vi "CameraSerialController_v06.vi"() -> (4 "图像时间戳":u32=16532020 format="%_32g")   [LabVIEW 2015]
uses:
  <vilib>/Instr/_visa.llb/VISA Configure Serial Port (Instr).vi
  MVCAMSDK.dll
  <vilib>/Analysis/NI_AALBase.lvlib
panel:
  in  "转动前进":T1=TRUE
  out "光强图 4":dbl[](graph)
  out "variance 4":dbl caption="方差" format="%0.2f"
  out "光强图 3":dbl[](graph)
  out "variance 3":dbl caption="方差" format="%0.2f"
  out "转动信号曲线":cluster{"Locations":dbl[], "Amplitudes":dbl[]}[](graph)=[{"Locations"=array[750 elements], "Amplitudes"=array[749 elements]}, {"Locations"=[104.38621227921368, 258.3247060234782, 410.71523318402836, 562.6858730022967, 712.7065754646931], "Amplitudes"=[11153.698204083417, 10559.387052180104, 10974.865031894917, 10500.852817232146, 11059.763900010517]}, {"Locations"=[26.787398227992274, 182.39455189327623, 333.5517219531509, 488.1851999460032, 636.5270621135614], "Amplitudes"=[3284.809720018355, 2039.4564261182056, 3638.2587716464914, 3082.2730888167225, 4217.856016996603]}]
  in  "平移回退":T1=TRUE
  in  "转动回退":T1=TRUE
  in  "转动计数":u16
  in  "转动一次脉冲数":u16=20
  in  "平移一次脉冲数":u16=20
  in  "平移计数":u16
  out "variance 2":dbl caption="方差" format="%0.2f"
  in  "flow control (0:none)":u16(ring) caption="流控制（0:无）" items=["无", "XON/XOFF", "RTS/CTS", "XON/XOFF & RTS/CTS", "DTR/DSR", "XON/XOFF & DTR/DSR"]
  in  "stop bits (10: 1 bit)":u16=10 caption="停止位（10: 1位）"
  in  "奇偶 (0:none)":enum16{"None", "Odd", "Even", "Mark", "Space"}(ring) caption="奇偶（0:无）"
  in  "数据比特(默认8)":u16(ring)=8 items=["5"=5, "6"=6, "7"=7, "8"=8]
  in  "波特率(默认9600)":u32=9600
  in  "端口":refnum<visa-resource-name>="COM1"
  in  "开始":T1=TRUE
  out "泰伯距离数值":dbl[](array[numeric])=[15.393849374426454, 15.239052716055017, 15.197063981826837, 15.002070246239633]
  out "Locations":dbl[](array[numeric])=[10.438621227921368, 25.832470602347822, 41.07152331840284, 56.268587300229676, 71.27065754646931] caption="上面图像曲线波峰位置"
  out "平移信号曲线":cluster{"Locations":dbl[], "Amplitudes":dbl[]}[](graph)=[{"Locations"=array[750 elements], "Amplitudes"=array[749 elements]}, {"Locations"=[104.38621227921368, 258.3247060234782, 410.71523318402836, 562.6858730022967, 712.7065754646931], "Amplitudes"=[11153.698204083417, 10559.387052180104, 10974.865031894917, 10500.852817232146, 11059.763900010517]}, {"Locations"=[26.787398227992274, 182.39455189327623, 333.5517219531509, 488.1851999460032, 636.5270621135614], "Amplitudes"=[3284.809720018355, 2039.4564261182056, 3638.2587716464914, 3082.2730888167225, 4217.856016996603]}]
  out "光强图 2":dbl[](graph)
  out "variance":dbl caption="方差" format="%0.2f"
  out "相机图像":T2(plugin-control)
  out "光强图":dbl[](graph)
  in  "自定义分辨率设置":bool
  in  "ROI分辨率":T3
  in  "预设分辨率设置":bool
  in  "预设分辨率":T4(radio)
  out "帧速":u32
  out "帧间耗时\n单位：（0.1ms）":u32
  in  "相机枚举":T5(ring)
  in  "自动曝光模式":bool=TRUE caption="软触发"
  in  "手动曝光模式":bool caption="软触发"
  in  "曝光时间，单位微秒":dbl=11000.0 format="%#_6f"
  in  "硬触发模式":bool caption="软触发"
  in  "软触发模式":bool caption="软触发"
  in  "连续模式":bool caption="软触发"
  in  "软触发一帧":bool caption="软触发"
  in  "读取自定义数据":bool
  out "从相机中读出的字符串(32字节)":string
  in  "写入自定义数据":bool
  in  "要写入相机的字符串(32字节)":string
  in  "拍照":bool
  in  "相机参数":bool=TRUE
  in  "Stop":bool
  in  "激活预览":bool=TRUE
  out "Image":T2(plugin-control)
  # "相机原生分辨率设置"
  # "写入自定义数据"
  # "触发设置"
  # "曝光设置"
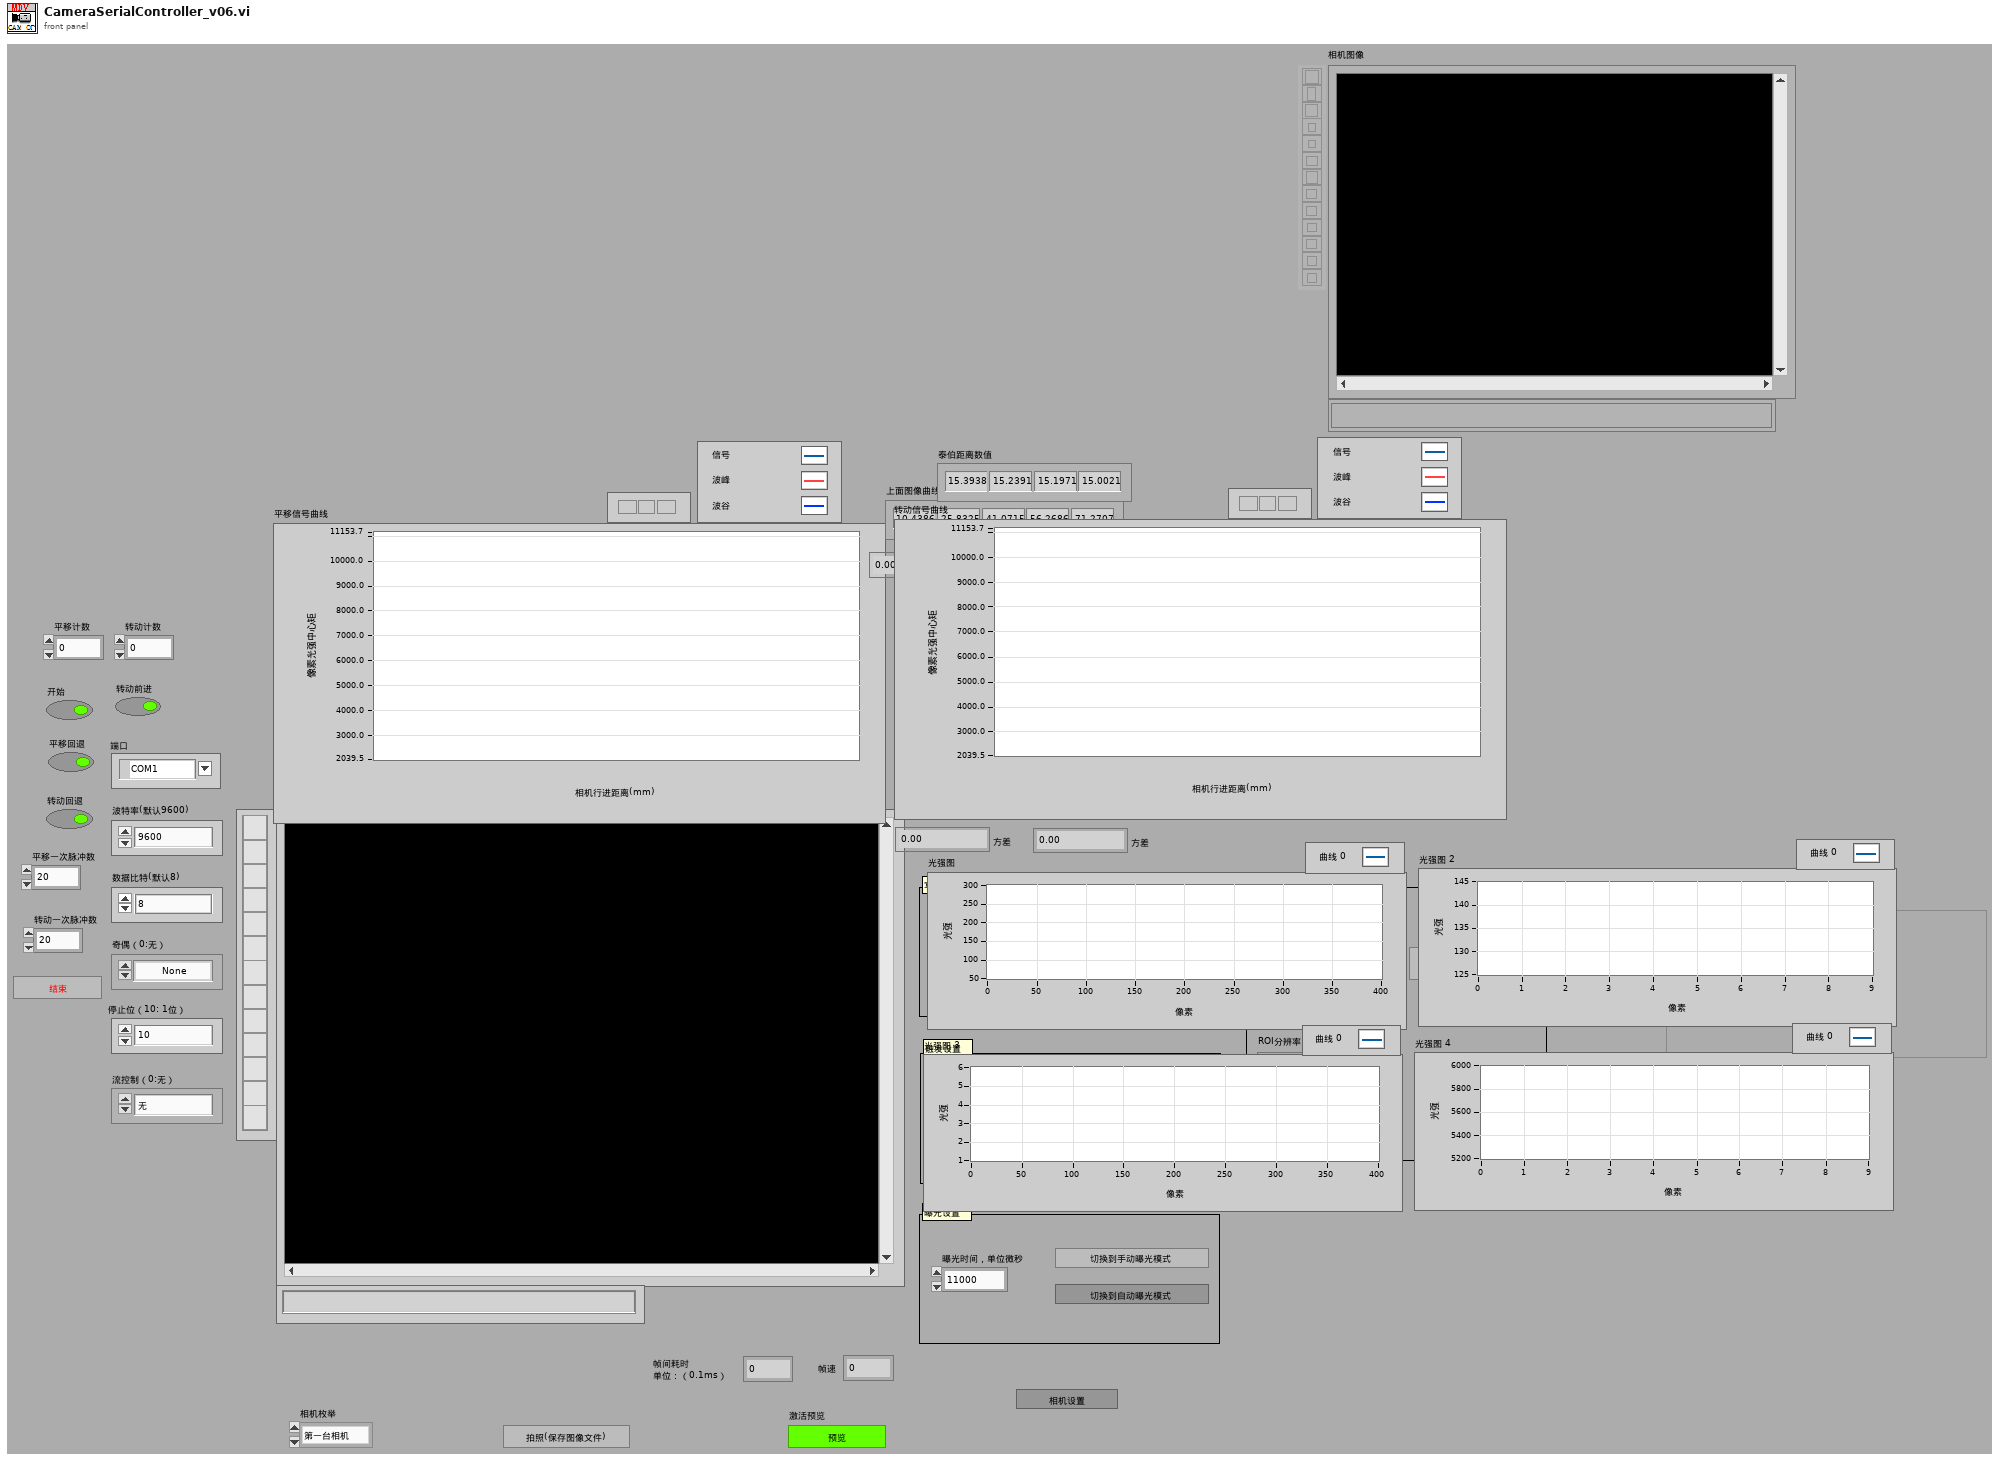
[diagram p1: front panel]
types:
  T1 = typedef "控件 1.ctl" = bool
  T2 = typedef "IMAQ Image.ctl" = refnum<image>
  T3 = cluster{"水平偏移":dbl, "垂直偏移":dbl, "宽度":dbl, "高度":dbl}
  T4 = enum32{"分辨率1", "分辨率2", "分辨率3", "分辨率4", "分辨率5", "分辨率6"}
  T5 = enum16{"第一台相机", "第二台相机", "第三台相机", "第四台相机", "第五台相机"}
  T6 = typedef "Image Type" = u32
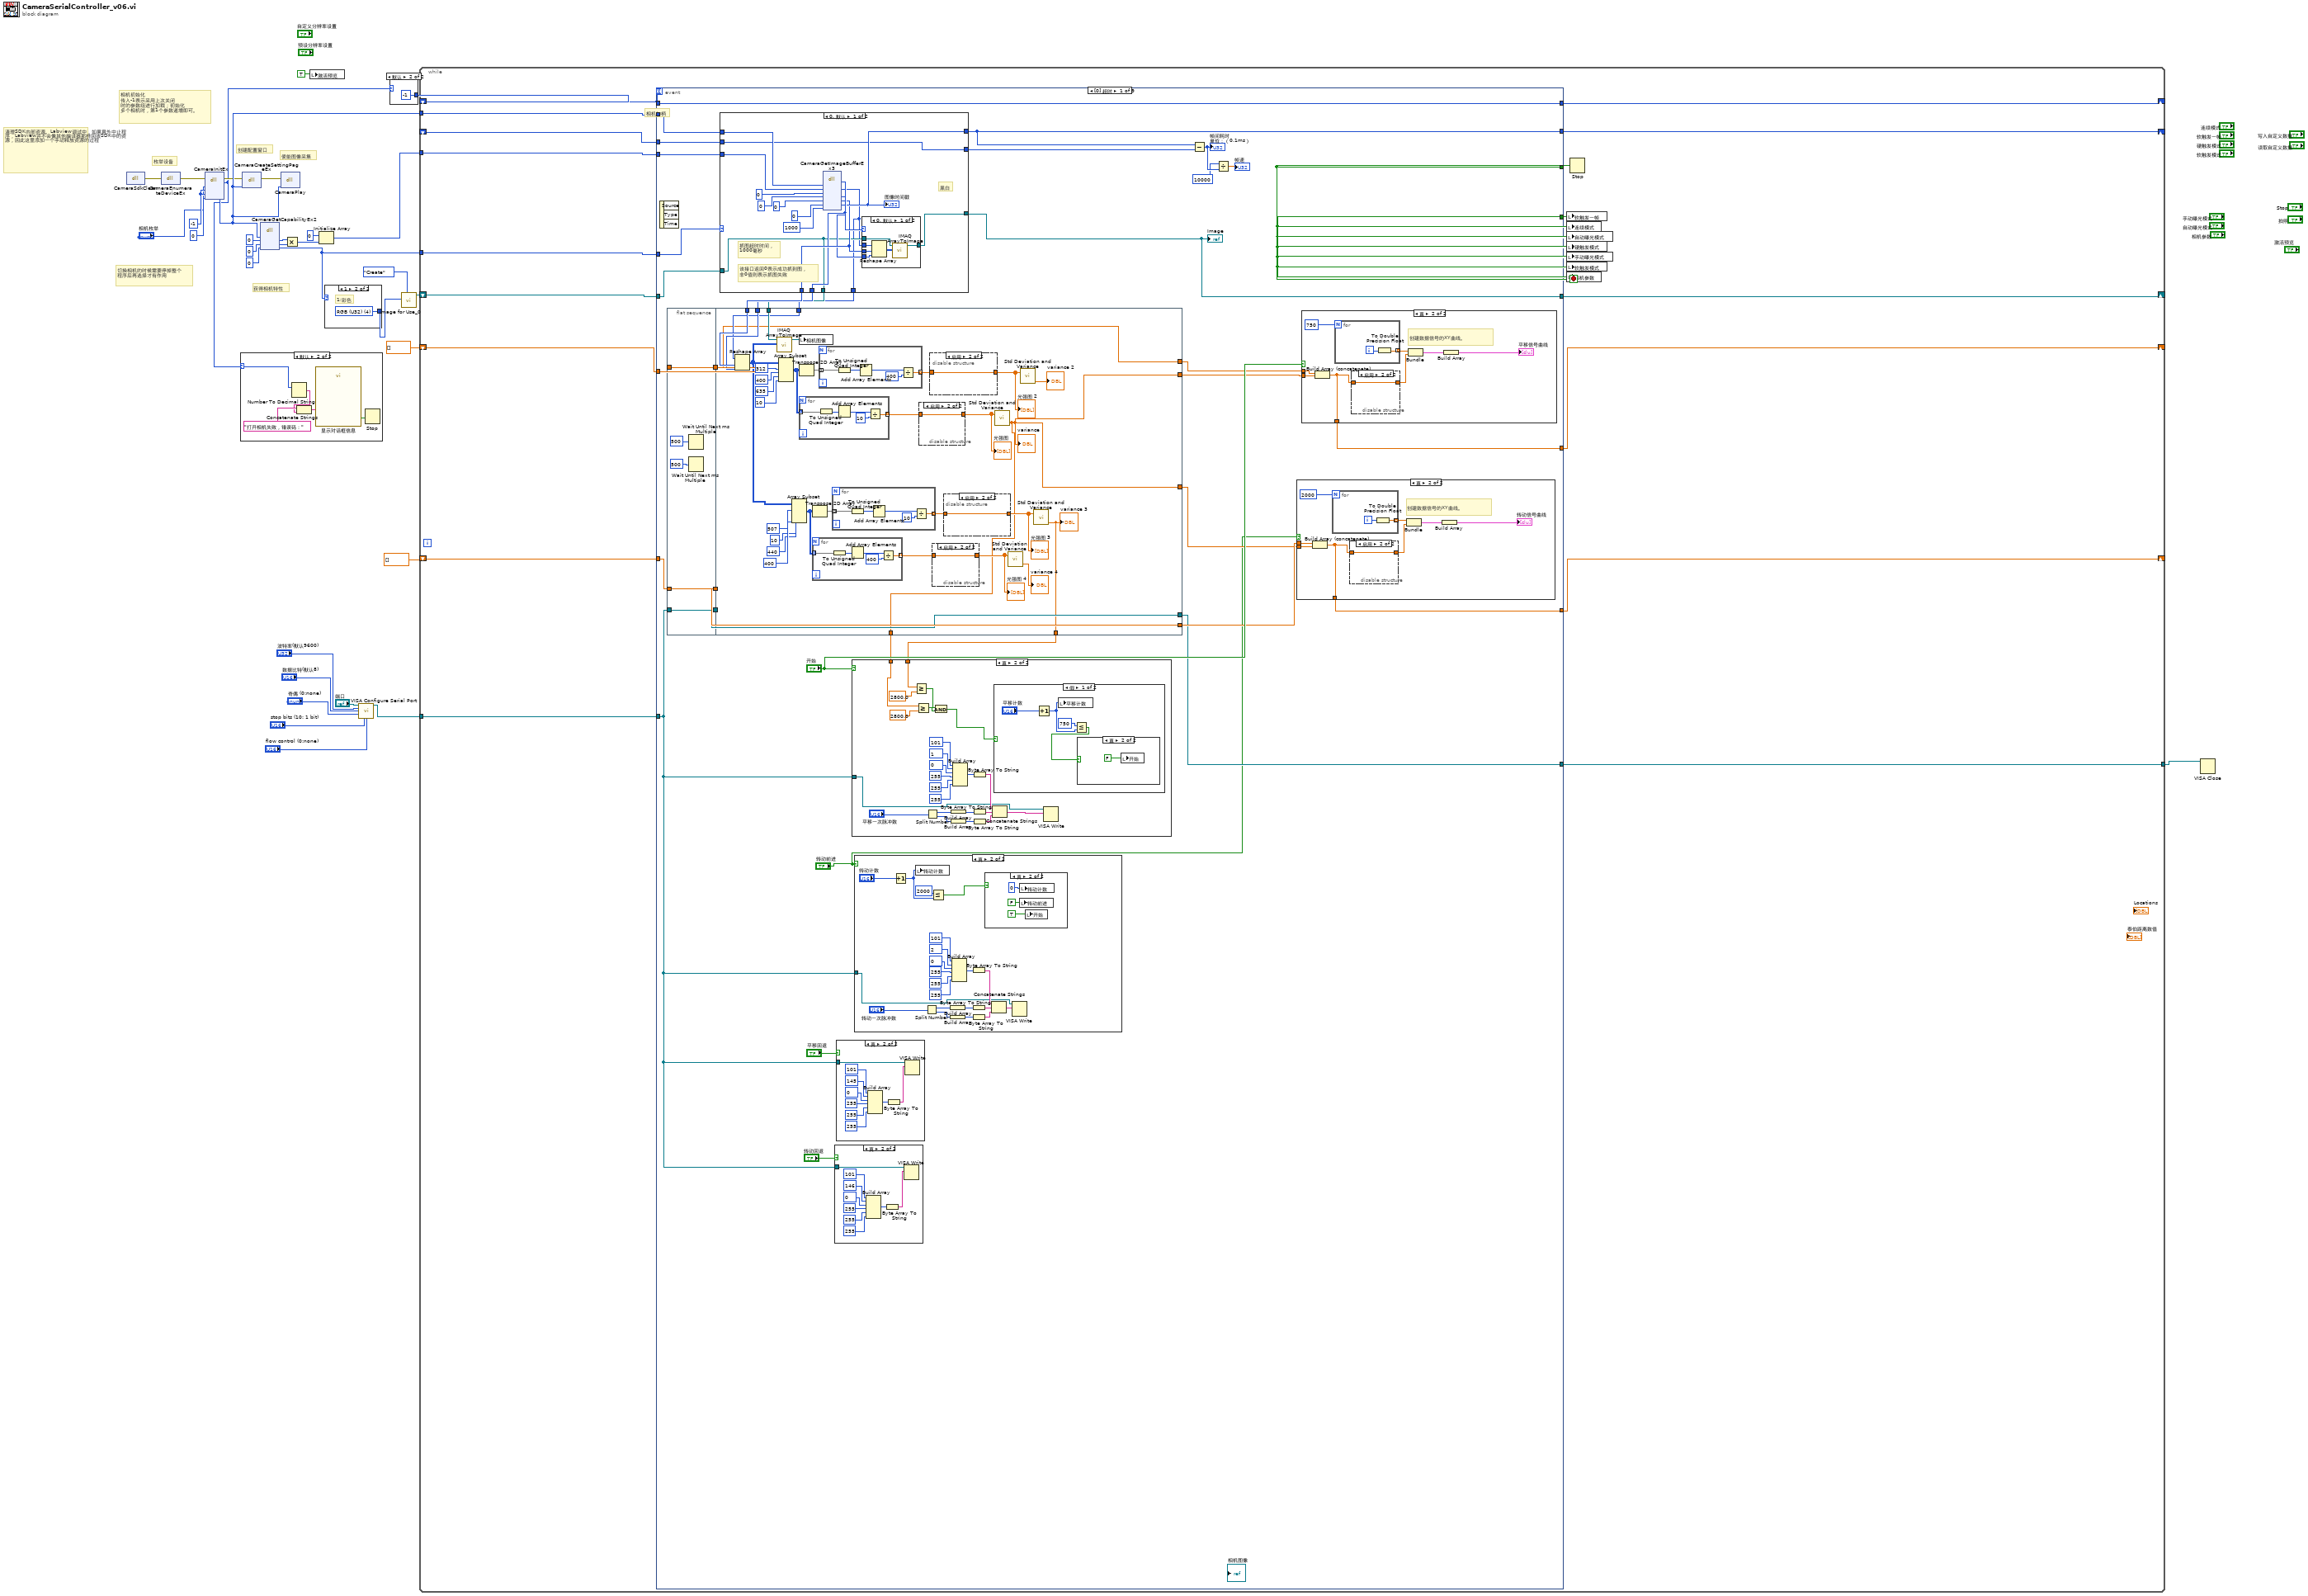
[diagram p0: block diagram]
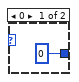
[diagram p2: hidden frame]
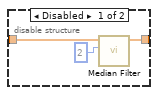
[diagram p4: hidden frame]
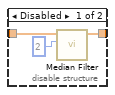
[diagram p5: hidden frame]
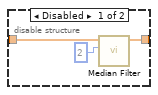
[diagram p6: hidden frame]
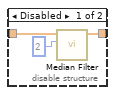
[diagram p7: hidden frame]
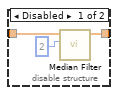
[diagram p9: hidden frame]
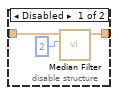
[diagram p11: hidden frame]
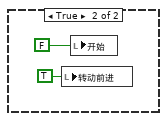
[diagram p18: hidden frame]
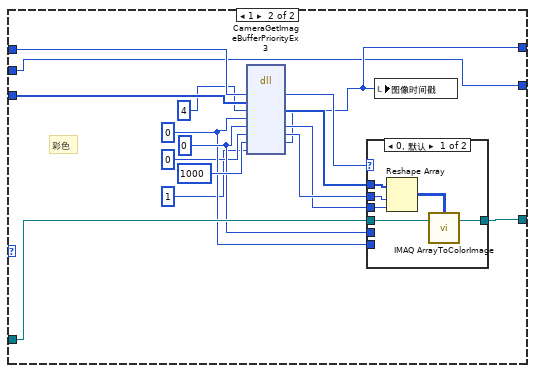
[diagram p20: hidden frame]
diagram:
  w30 = -1
  # "切换相机的时候需要停掉整个\n程序后再选择才有作用"
  # "清理SDK内部资源。Labview调试中，如果意外中止程序，Labview并不会像其他编译器那样回收SDK中的资源，因此这里添加一个手动释放资源的过程"
  # "使能图像采集"
  # "获得相机特性"
  # "创建配置窗口"
  # "相机初始化\n传入-1表示采用上次关闭\n时的参数组进行加载；初始化\n多个相机时，第1个参数递增即可。"
  # "枚举设备"
  n1 = dll-call lib="MVCAMSDK.dll" fn="CameraSdkClean"() -> (error out=w31:errorcluster)  [unwired: 4 in, 1 out]
  n2 = dll-call lib="MVCAMSDK.dll" fn="CameraEnumerateDeviceEx"(error in=w31) -> (error out=w28:errorcluster)  [unwired: 3 in, 1 out]
  n3 = dll-call lib="MVCAMSDK.dll" fn="CameraInitEx"(error in=w28, "相机索引值"="相机枚举", "参数加载方式"=w30, "要加载的参数组索引"=w30, "相机句柄"=0) -> (error out=w17:errorcluster, "返回类型"=w12:i32, "相机句柄"=w19:i32)  [unwired: 5 in, 1 out]
  n4 = case shown="默认" w12 {
    selector: w12 -> [_ w37]
    frame 0 {
    }
    frame Default {
      n5 = Number To Decimal String(number=w37) -> (decimal integer string=w34:string)  [unwired: 1 in]
      n6 = Concatenate Strings("打开相机失败，错误码：" ("字符串"), w34) -> (w36:string)
      n7 = call "显示对话框信息"("Message"=w36) -> ("结束"=w38:bool)  [unwired: 9 in, 1 out]
      n8 = Stop(stop? (T)=w38) -> ()
    }
  }
  n9 = dll-call lib="MVCAMSDK.dll" fn="CameraCreateSettingPageEx"(error in=w17, "相机句柄"=w19) -> (error out=w20:errorcluster)  [unwired: 4 in, 1 out]
  n10 = dll-call lib="MVCAMSDK.dll" fn="CameraGetCapabilityEx2"("相机句柄"=w19, "图像最大宽度"=0, "图像最大高度"=0, "是否是彩色相机(返回0:黑白;1:彩色)"=0) -> ("图像最大宽度"=w22:i32, "图像最大高度"=w21:i32, "是否是彩色相机(返回0:黑白;1:彩色)"=w16:i32)  [unwired: 5 in, 2 out]
  n11 = dll-call lib="MVCAMSDK.dll" fn="CameraPlay"(error in=w20, "相机句柄"=w19) -> ()  [unwired: 4 in, 2 out]
  n12 = Multiply(x=w22, y=w21) -> (x*y=w26:i32)
  n13 = local write "激活预览"(TRUE ("激活预览")) -> ()
  n14 = Initialize Array(0, w26) -> (w18:i32[])
  n15 = case shown="1" w16 {
    tunnel: [_ w39] -> w32
    frame 0, Default {
      # "0:黑白;"
    }
    frame 1 {
      w39 = T6 4 items=["Grayscale (U8)", "Grayscale (I16)", "Grayscale (SGL)", "Complex (CSG)", "RGB (U32)", "HSL (U32)", "RGB (U64)", "Grayscale (U16)"] ("Image Type")
      # "1:彩色"
    }
  }
  n16 = call-poly "VISA Configure Serial Port"("VISA resource name"="端口", "baud rate (9600)"="波特率(默认9600)", "data bits (8)"="数据比特(默认8)", "parity (0:none)"="奇偶 (0:none)", "stop bits (10: 1 bit)"="stop bits (10: 1 bit)", "flow control (0:none)"="flow control (0:none)") -> ("VISA resource name out"=w4:refnum<visa-resource-name>)  [unwired: 8 in, 1 out]
  n17 = case shown="默认" w12 {
    tunnel: [0 -1] -> w11
    frame 0 {
    }
    frame Default {
    }
  }
  n18 = call "Image for Use_0.vi"("Command"=enum16{"Create", "Use", "Copy in", "Dispose"}."Create", "Image Type"=w32) -> ("Image out"=w15:T2)  [unwired: 8 in, 1 out]
  n19 = while {
    tunnel: w19 -> [w55]
    tunnel: w18 -> [w57]
    tunnel: w16 -> [w58]
    shift-right: [w54] -> _
    shift-left: w11 -> [w53]
    shift-right: [w51] -> _
    shift-left: w15 -> [w56]
    shift-right: [w50] -> _
    shift-left: _ -> [w49]
    tunnel: w4 -> [w47]
    tunnel: [w46] -> w3
    shift-right: [w44] -> _
    shift-left: dbl[] [] -> [w45]
    shift-right: [w43] -> _
    shift-left: dbl[] [] -> [w42]
    stop <- w48 stop-if-true
    # "相机句柄"
    n20 = event shown="[0] 超时" {
      selector: _ -> [_ _ _ _ _ _ _ _ _]
      dyn-events: _ -> [_ _ _ _ _ _ _ _ _]
      timeout: w53 -> [_ _ _ _ _ _ _ _ _]
      tunnel: [_ _ _ _ _ _ _ _ TRUE] -> w48
      tunnel: w57 -> [w92 _ _ _ _ _ _ _ _]
      tunnel: w58 -> [w91 _ _ _ _ _ _ _ _]
      tunnel: w55 -> [w93 _ w324 w342 w357 _ w371 w394 w474]
      tunnel: w56 -> [w90 w317 w323 w341 w356 w361 w370 w396 w472]
      tunnel: [w89 w318 w325 w343 w358 w362 w372 w397 w475] -> w54
      tunnel: w53 -> [w89 _ w325 w343 w358 w362 w372 w397 w475]
      tunnel: [_ _ _ _ _ _ _ _ FALSE] -> w52
      tunnel: [w88 w317 w323 w341 w356 w361 w370 w396 w472] -> w51
      tunnel: [w85 w316 w322 w340 w355 w360 w369 w388 w471] -> w50
      tunnel: w49 -> [w87 w316 w322 w340 w355 w360 w369 w388 w471]
      tunnel: w47 -> [w66 _ _ _ _ _ _ _ _]
      tunnel: [w65 _ _ _ _ _ _ _ _] -> w46
      tunnel: w45 -> [w72 _ _ _ _ _ _ _ _]
      tunnel: [w74 _ _ _ _ _ _ _ _] -> w44
      tunnel: [w73 _ _ _ _ _ _ _ _] -> w43
      tunnel: w42 -> [w68 _ _ _ _ _ _ _ _]
      event Timeout {
        n21 = event-data() -> ()  [unwired: 1 in, 3 out]
        n22 = flat-sequence {
          tunnel: w72 -> [w98]
          tunnel: [w98] -> w71
          tunnel: [w95] -> w69
          tunnel: w68 -> [w95]
          tunnel: [w94] -> w67
          tunnel: w66 -> [w94]
          tunnel: w81 -> [w130]
          tunnel: w80 -> [w129]
          tunnel: w79 -> [w128]
          tunnel: w78 -> [w127]
          tunnel: [w99] -> w63
          tunnel: [w116] -> w62
          tunnel: w71 -> [w116]
          tunnel: [w115] -> w70
          tunnel: w69 -> [w115]
          tunnel: [w114] -> w65
          tunnel: w67 -> [w114]
          tunnel: [w99] -> w64
          tunnel: [w100] -> w61
          tunnel: [w99] -> w60
          frame #0 {
            n23 = Wait Until Next ms Multiple(millisecond multiple=u32 500 ("毫秒倍数")) -> ()  [unwired: 1 out]
            n24 = Wait Until Next ms Multiple(millisecond multiple=u32 500 ("毫秒倍数")) -> ()  [unwired: 1 out]
          }
          frame #1 {
            n25 = Reshape Array(w127, w130, w129) -> (w101:u8[][])
            n26 = call "IMAQ ArrayToImage"("Image Pixels (U8)"=w101, "Image"=w128) -> ("Image Out"=w131:T2)  [unwired: 8 in, 1 out]
            n27 = Array Subset(array=w101, index (row)=312 ("索引"), length (row)=400 ("长度"), index (col)=635 ("长度"), length (col)=10 ("索引")) -> (w117:u8[][])
            n28 = Array Subset(array=w101, index (row)=507 ("索引"), length (row)=10 ("长度"), index (col)=440 ("长度"), length (col)=400 ("索引")) -> (w112:u8[][])
            n29 = local write "相机图像"(w131) -> ()
            n30 = Transpose 2D Array(2D array=w117) -> (transposed array=w124:u8[][])
            n31 = for {
              tunnel: w117 -> [w162] mode=indexing
              tunnel: [w160] -> w126 mode=indexing
              n32 = To Unsigned Quad Integer(1:w162) -> (0:w161:u64[])
              n33 = Add Array Elements(numeric array=w161) -> (sum=w163:u64)
              n34 = Divide(x=w163, y=u64 10) -> (x/y=w160:dbl)
            }
            n35 = Transpose 2D Array(2D array=w112) -> (transposed array=w105:u8[][])
            n36 = for {
              tunnel: w112 -> [w144] mode=indexing
              tunnel: [w142] -> w103 mode=indexing
              n37 = To Unsigned Quad Integer(1:w144) -> (0:w143:u64[])
              n38 = Add Array Elements(numeric array=w143) -> (sum=w145:u64)
              n39 = Divide(x=w145, y=u64 400) -> (x/y=w142:dbl)
            }
            n40 = for {
              tunnel: w124 -> [w153] mode=indexing
              tunnel: [w151] -> w125 mode=indexing
              n41 = To Unsigned Quad Integer(1:w153) -> (0:w152:u64[])
              n42 = Add Array Elements(numeric array=w152) -> (sum=w154:u64)
              n43 = Divide(x=w154, y=u64 400) -> (x/y=w151:dbl)
            }
            n44 = for {
              tunnel: w105 -> [w135] mode=indexing
              tunnel: [w133] -> w104 mode=indexing
              n45 = To Unsigned Quad Integer(1:w135) -> (0:w134:u64[])
              n46 = Add Array Elements(numeric array=w134) -> (sum=w136:u64)
              n47 = Divide(x=w136, y=u64 10) -> (x/y=w133:dbl)
            }
            n48 = disable-structure shown="启用" {
              disable-tunnel: w126 -> [w166 w167]
              disable-tunnel: [w164 w167] -> w123
              frame Disabled {
                n49 = call <vilib>:"Median Filter.vi"("left rank"=2, "X"=w166) -> ("Filtered X"=w164:dbl[])  [unwired: 8 in, 1 out]
              }
              frame Enabled {
              }
            }
            "光强图" <- w123
            n50 = disable-structure shown="启用" {
              disable-tunnel: w125 -> [w157 w158]
              disable-tunnel: [w155 w158] -> w122
              frame Disabled {
                n51 = call <vilib>:"Median Filter.vi"("left rank"=2, "X"=w157) -> ("Filtered X"=w155:dbl[])  [unwired: 8 in, 1 out]
              }
              frame Enabled {
              }
            }
            "光强图 2" <- w122
            n52 = disable-structure shown="启用" {
              disable-tunnel: w103 -> [w148 w149]
              disable-tunnel: [w146 w149] -> w106
              frame Disabled {
                n53 = call <vilib>:"Median Filter.vi"("left rank"=2, "X"=w148) -> ("Filtered X"=w146:dbl[])  [unwired: 8 in, 1 out]
              }
              frame Enabled {
              }
            }
            "光强图 4" <- w106
            n54 = disable-structure shown="启用" {
              disable-tunnel: w104 -> [w139 w140]
              disable-tunnel: [w137 w140] -> w107
              frame Disabled {
                n55 = call <vilib>:"Median Filter.vi"("left rank"=2, "X"=w139) -> ("Filtered X"=w137:dbl[])  [unwired: 8 in, 1 out]
              }
              frame Enabled {
              }
            }
            "光强图 3" <- w107
            n56 = call <vilib>:"Std Deviation and Variance.vi"("X"=w123) -> ("variance"=w99:dbl)  [unwired: 1 in, 2 out]
            "variance" <- w99
            n57 = call <vilib>:"Std Deviation and Variance.vi"("X"=w106) -> ("variance"=→"variance 4":dbl)  [unwired: 1 in, 2 out]
            n58 = call <vilib>:"Std Deviation and Variance.vi"("X"=w122) -> ("variance"=→"variance 2":dbl)  [unwired: 1 in, 2 out]
            n59 = call <vilib>:"Std Deviation and Variance.vi"("X"=w107) -> ("variance"=w100:dbl)  [unwired: 1 in, 2 out]
            "variance 3" <- w100
          }
        }
        n60 = case shown="0, 默认" w91 {
          tunnel: w92 -> [w285 w308]
          tunnel: w90 -> [w272 w307]
          tunnel: w93 -> [w277 w306]
          tunnel: [w278 w296] -> w88
          tunnel: [w276 w295] -> w85
          tunnel: w87 -> [w275 w294]
          tunnel: [w275 w294] -> w86
          tunnel: [w274 _] -> w81
          tunnel: [w273 _] -> w80
          tunnel: [w272 _] -> w79
          tunnel: [w271 _] -> w78
          frame 0, Default {
            # "黑白"
            # "该接口返回0表示成功抓到图，\n非0值则表示抓图失败"
            # "抓图超时时间，\n1000毫秒"
            n61 = dll-call lib="MVCAMSDK.dll" fn="CameraGetImageBufferEx3"("相机句柄"=w277, "图像数据缓冲区"=w285, "图像输出格式(0:8位灰度;1:24位彩色;2:32位彩色，3：BGR24彩色 4：BGRA32位彩色)"=0, "图像宽度"=0, "图像高度"=0, "时间戳(单位为100微秒)"=0, "抓图超时时间(毫秒)"=1000) -> ("返回类型"=w280:i32, "图像数据缓冲区"=w271:u8[], "图像宽度"=w273:i32, "图像高度"=w274:i32, "时间戳(单位为100微秒)"=w276:u32)  [unwired: 6 in, 2 out]
            "图像时间戳" <- w276
            n62 = case shown="0, 默认" w280 {
              tunnel: w271 -> [w291 _]
              tunnel: w272 -> [w288 w292]
              tunnel: w274 -> [w290 _]
              tunnel: w273 -> [w289 _]
              tunnel: [w286 w292] -> w278
              frame 0, Default {
                n63 = Reshape Array(w291, w290, w289) -> (w287:u8[][])
                n64 = call "IMAQ ArrayToImage"("Image Pixels (U8)"=w287, "Image"=w288) -> ("Image Out"=w286:T2)  [unwired: 8 in, 1 out]
              }
              frame -12 {
              }
            }
          }
          frame 1 {
            w298 = 0
            w299 = 0
            # "彩色"
            n65 = dll-call lib="MVCAMSDK.dll" fn="CameraGetImageBufferPriorityEx3"("相机句柄"=w306, "图像数据缓冲区"=w308, "图像输出格式(0:8位灰度;1:24位彩色;2:32位彩色)"=4, "图像宽度"=w298, "图像高度"=w299, "时间戳（单位为100微秒）"=0, "抓图超时时间(毫秒)"=1000, "取图优先级(0: 取最旧   1:取最新)"=1) -> ("返回类型"=w300:i32, "图像数据缓冲区"=w303:u32[], "图像宽度"=w301:i32, "图像高度"=w302:i32, "时间戳（单位为100微秒）"=w295:u32)  [unwired: 7 in, 2 out]
            n66 = case shown="0, 默认" w300 {
              tunnel: w303 -> [w313 _]
              tunnel: w307 -> [w312 w315]
              tunnel: w302 -> [w311 _]
              tunnel: w301 -> [w310 _]
              tunnel: w299 -> [_ _]
              tunnel: w298 -> [_ _]
              tunnel: [w309 w315] -> w296
              frame 0, Default {
                n67 = Reshape Array(w313, w311, w310) -> (w314:u32[][])
                n68 = call "IMAQ ArrayToColorImage"("Image Pixels (U32)"=w314, "Image"=w312) -> ("Image Out"=w309:T2)  [unwired: 3 in, 1 out]
              }
              frame -12 {
              }
            }
            n69 = local write "图像时间戳"(w295) -> ()
          }
        }
        "Image" <- w88
        n70 = case shown="真" "转动回退" {
          tunnel: w66 -> [_ w199]
          frame False {
          }
          frame True {
            n71 = Build Array(101, 146, 0, 255, 255, 255) -> (w200:i32[])
            n72 = Byte Array To String(unsigned byte array=w200) -> (string=w198:string)
            n73 = VISA Write(VISA resource name=w199, write buffer=w198) -> ()  [unwired: 1 in, 3 out]
          }
        }
        n74 = case shown="真" "平移回退" {
          tunnel: w66 -> [_ w208]
          frame False {
          }
          frame True {
            n75 = Build Array(101, 145, 0, 255, 255, 255) -> (w209:i32[])
            n76 = Byte Array To String(unsigned byte array=w209) -> (string=w207:string)
            n77 = VISA Write(VISA resource name=w208, write buffer=w207) -> ()  [unwired: 1 in, 3 out]
          }
        }
        n78 = case shown="真" "开始" {
          tunnel: w66 -> [_ w248]
          tunnel: w61 -> [_ w246]
          tunnel: w60 -> [_ w245]
          frame False {
          }
          frame True {
            n79 = Greater Or Equal?(x=w246, y=2800.0) -> (x >= y?=w242:bool)
            n80 = Greater Or Equal?(x=w245, y=2800.0) -> (x >= y?=w241:bool)
            n81 = Split Number(x="平移一次脉冲数") -> (hi(x)=w256:u8, lo(x)=w255:u8)
            n82 = And(x=w242, y=w241) -> (x .and. y?=w240:bool)
            n83 = Build Array(w256) -> (w254:u8[])
            n84 = Build Array(w255) -> (w253:u8[])
            n85 = Build Array(101, 1, 0, 255, 255, 255) -> (w252:i32[])
            n86 = Byte Array To String(unsigned byte array=w252) -> (string=w251:string)
            n87 = Byte Array To String(unsigned byte array=w254) -> (string=w250:string)
            n88 = Byte Array To String(unsigned byte array=w253) -> (string=w249:string)
            n89 = Concatenate Strings(w251, w250, w249) -> (w247:string)
            n90 = case shown="假" w240 {
              frame False {
                n91 = Increment(x="平移计数") -> (x+1=w265:u16)
                n92 = local write "平移计数"(w265) -> ()
                n93 = Less Or Equal?(x=750, y=w265) -> (x <= y?=w264:bool)
                n94 = case shown="真" w264 {
                  frame False {
                  }
                  frame True {
                    n95 = local write "开始"(T1 FALSE ("平移前进")) -> ()
                  }
                }
              }
              frame True {
                n96 = local write "转动前进"(T1 TRUE ("平移前进")) -> ()
                n97 = local write "开始"(T1 FALSE ("平移前进")) -> ()
              }
            }
            n98 = VISA Write(VISA resource name=w248, write buffer=w247) -> ()  [unwired: 1 in, 3 out]
          }
        }
        n99 = case shown="真" "转动前进" {
          tunnel: w66 -> [_ w220]
          frame False {
          }
          frame True {
            n100 = Increment(x="转动计数") -> (x+1=w218:u16)
            n101 = local write "转动计数"(w218) -> ()
            n102 = Split Number(x="转动一次脉冲数") -> (hi(x)=w228:u8, lo(x)=w227:u8)
            n103 = Less Or Equal?(x=2000, y=w218) -> (x <= y?=w230:bool)
            n104 = Build Array(w228) -> (w226:u8[])
            n105 = Build Array(w227) -> (w225:u8[])
            n106 = Build Array(101, 2, 0, 255, 255, 255) -> (w224:i32[])
            n107 = Byte Array To String(unsigned byte array=w224) -> (string=w223:string)
            n108 = Byte Array To String(unsigned byte array=w226) -> (string=w222:string)
            n109 = Byte Array To String(unsigned byte array=w225) -> (string=w221:string)
            n110 = case shown="真" w230 {
              frame False {
              }
              frame True {
                n111 = local write "转动前进"(T1 FALSE ("平移前进")) -> ()
                n112 = local write "转动计数"(u16 0 ("平移计数")) -> ()
                n113 = local write "开始"(T1 TRUE ("平移前进")) -> ()
              }
            }
            n114 = Concatenate Strings(w223, w222, w221) -> (w217:string)
            n115 = VISA Write(VISA resource name=w220, write buffer=w217) -> ()  [unwired: 1 in, 3 out]
          }
        }
        n116 = Subtract(x=w85, y=w86) -> (x-y=w84:u32)
        "帧间耗时\n单位：（0.1ms）" <- w84
        n117 = Divide(x=u32 10000 ("帧间耗时"), y=w84) -> (x/y=→"帧速":dbl)
        n118 = case shown="真" "转动前进" {
          tunnel: w64 -> [_ w171]
          tunnel: w70 -> [w168 w170]
          tunnel: [w168 w169] -> w73
          frame False {
          }
          frame True {
            # "创建数据信号的XY曲线。"
            n119 = Build Array (concatenate)(w170, w171) -> (w169:dbl[])
            n120 = for {
              N: i64 2000 ("数值") -> [_]
              tunnel: [w177] -> w173 mode=indexing
              i -> [w178]
              n121 = To Double Precision Float(number=w178) -> (double precision float=w177:dbl)
            }
            n122 = disable-structure shown="启用" {
              disable-tunnel: w169 -> [w180 w182]
              disable-tunnel: [w179 w182] -> w174
              frame Disabled {
                n123 = call <vilib>:"Median Filter.vi"("left rank"=2, "X"=w180) -> ("Filtered X"=w179:dbl[])  [unwired: 8 in, 1 out]
              }
              frame Enabled {
              }
            }
            n124 = Bundle(w173, w174) -> (w176:cluster{dbl[], dbl[]})  [unwired: 1 in]
            n125 = Build Array(w176) -> (→"转动信号曲线":cluster{dbl[], dbl[]}[])
          }
        }
        n126 = case shown="真" "开始" {
          tunnel: w62 -> [w183 w185]
          tunnel: w63 -> [_ w186]
          tunnel: [w183 w184] -> w74
          frame False {
          }
          frame True {
            # "创建数据信号的XY曲线。"
            n127 = Build Array (concatenate)(w185, w186) -> (w184:dbl[])
            n128 = for {
              N: i64 750 ("数值") -> [_]
              tunnel: [w192] -> w190 mode=indexing
              i -> [w193]
              n129 = To Double Precision Float(number=w193) -> (double precision float=w192:dbl)
            }
            n130 = disable-structure shown="启用" {
              disable-tunnel: w184 -> [w195 w197]
              disable-tunnel: [w194 w197] -> w189
              frame Disabled {
                n131 = call <vilib>:"Median Filter.vi"("left rank"=2, "X"=w195) -> ("Filtered X"=w194:dbl[])  [unwired: 8 in, 1 out]
              }
              frame Enabled {
              }
            }
            n132 = Bundle(w190, w189) -> (w187:cluster{dbl[], dbl[]})  [unwired: 1 in]
            n133 = Build Array(w187) -> (→"平移信号曲线":cluster{dbl[], dbl[]}[])
          }
        }
      }
      event "激活预览": Value Change {
        n134 = event-data() -> ("NewVal"=w319:bool)  [unwired: 1 in, 5 out]
        n135 = case shown="真" w319 {
          tunnel: [-1 0] -> w318
          frame False {
          }
          frame True {
          }
        }
      }
      event "连续模式", "软触发一帧", "硬触发模式", "软触发模式": Value Change {
        n136 = event-data() -> ("CtlRef"=w327:refnum<vi>)  [unwired: 1 in, 5 out]
        n137 = control-ref of="连续模式"() -> (w329:refnum<vi>)
        n138 = control-ref of="硬触发模式"() -> (w330:refnum<vi>)
        n139 = control-ref of="软触发模式"() -> (w331:refnum<vi>)
        n140 = control-ref of="软触发一帧"() -> (w332:refnum<vi>)
        n141 = Build Array ("创建数组")(w329, w330, w331, w332) -> (w328:refnum<vi>[])
        n142 = Search 1D Array(1D array=w328, element=w327) -> (index of element=w326:i32)  [unwired: 1 in]
        n143 = case shown="1" w326 {
          tunnel: w324 -> [w333 w335 w337 w339]
          frame 0, Default {
            # "连续模式"
            n144 = dll-call lib="MVCAMSDK.dll" fn="CameraSetTriggerMode"("相机句柄"=w333, "模式"=0) -> ()  [unwired: 6 in, 2 out]
          }
          frame 1 {
            # "硬触发模式"
            n145 = dll-call lib="MVCAMSDK.dll" fn="CameraSetTriggerMode"("相机句柄"=w335, "模式"=2) -> ()  [unwired: 6 in, 2 out]
          }
          frame 2 {
            # "软触发模式"
            n146 = dll-call lib="MVCAMSDK.dll" fn="CameraSetTriggerMode"("相机句柄"=w337, "模式"=1) -> ()  [unwired: 6 in, 2 out]
          }
          frame 3 {
            # "软触发一帧"
            n147 = dll-call lib="MVCAMSDK.dll" fn="CameraSoftTrigger"("相机句柄"=w339) -> ()  [unwired: 5 in, 2 out]
          }
        }
      }
      event "手动曝光模式", "自动曝光模式": Value Change {
        n148 = event-data() -> ("CtlRef"=w346:refnum<vi>)  [unwired: 1 in, 5 out]
        n149 = control-ref of="自动曝光模式"() -> (w344:refnum<vi>)
        n150 = control-ref of="手动曝光模式"() -> (w347:refnum<vi>)
        n151 = Build Array ("创建数组")(w347, w344) -> (w348:refnum<vi>[])
        n152 = Search 1D Array(1D array=w348, element=w346) -> (index of element=w345:i32)  [unwired: 1 in]
        n153 = case shown="0, 默认" w345 {
          tunnel: w342 -> [w349 w353]
          frame 0, Default {
            # "手动曝光模式"
            n154 = dll-call lib="MVCAMSDK.dll" fn="CameraSetAeState"("相机句柄"=w349, "曝光模式(0手动，1自动)"=0) -> (error out=w352:errorcluster)  [unwired: 6 in, 1 out]
            n155 = dll-call lib="MVCAMSDK.dll" fn="CameraSetExposureTime"(error in=w352, "相机句柄"=w349, "曝光时间，单位微秒"="曝光时间，单位微秒") -> ()  [unwired: 5 in, 2 out]
          }
          frame 1 {
            # "自动曝光模式"
            n156 = dll-call lib="MVCAMSDK.dll" fn="CameraSetAeState"("相机句柄"=w353, "曝光模式(0手动，1自动)"=1) -> ()  [unwired: 6 in, 2 out]
          }
        }
      }
      event "相机参数": Value Change {
        n157 = event-data() -> ()  [unwired: 1 in, 6 out]
        n158 = dll-call lib="MVCAMSDK.dll" fn="CameraShowSettingPage"("相机句柄"=w357, "状态"=TRUE) -> ()  [unwired: 6 in, 2 out]
      }
      event "拍照": Value Change {
        n159 = event-data() -> ()  [unwired: 1 in, 6 out]
        n160 = local read "Image"() -> (w363:T2)
        n161 = Format Date/Time String(time format string (%c)="%Y-%m-%d %H：%M：%S.bmp ") -> (date/time string=w367:string)  [unwired: 2 in]
        n162 = Concatenate Strings("c:\\", w367) -> (w364:string)
        n163 = String To Path(string=w364) -> (path=w366:path)
        n164 = call-poly "IMAQ Write File 2"("File Path"=w366, "Image"=w363) -> ()  [unwired: 8 in, 2 out]
      }
      event "写入自定义数据", "读取自定义数据": Value Change {
        n165 = event-data() -> ("CtlRef"=w374:refnum<vi>)  [unwired: 1 in, 5 out]
        n166 = control-ref of="读取自定义数据"() -> (w376:refnum<vi>)
        n167 = control-ref of="写入自定义数据"() -> (w375:refnum<vi>)
        n168 = Build Array ("创建数组")(w376, w375) -> (w377:refnum<vi>[])
        n169 = Search 1D Array(1D array=w377, element=w374) -> (index of element=w373:i32)  [unwired: 1 in]
        n170 = case shown="0, 默认" w373 {
          tunnel: w371 -> [w378 w385]
          frame 0, Default {
            n171 = Initialize Array(0, 32) -> (w382:i32[])
            n172 = dll-call lib="MVCAMSDK.dll" fn="CameraReadSN"("相机句柄"=w378, "序列号"=w382, "序列号级别，[0,1,2],0级为只读，1,2级可写"=1) -> ("序列号"=w380:u8[])  [unwired: 6 in, 2 out]
            n173 = Byte Array To String(unsigned byte array=w380) -> (string=→"从相机中读出的字符串(32字节)":string)
          }
          frame 1 {
            n174 = dll-call lib="MVCAMSDK.dll" fn="CameraWriteSN"("相机句柄"=w385, "序列号(固定为32个字节)"="要写入相机的字符串(32字节)", "序列号级别，[0,1,2]对应3级序列号，其中0级为只读，1,2级可写"=1) -> ()  [unwired: 7 in, 2 out]
          }
        }
      }
      event "预设分辨率设置", "自定义分辨率设置": Value Change {
        n175 = event-data() -> ("CtlRef"=w390:refnum<vi>)  [unwired: 1 in, 5 out]
        n176 = control-ref of="预设分辨率设置"() -> (w392:refnum<vi>)
        n177 = control-ref of="自定义分辨率设置"() -> (w391:refnum<vi>)
        n178 = Build Array ("创建数组")(w392, w391) -> (w393:refnum<vi>[])
        n179 = Search 1D Array(1D array=w393, element=w390) -> (index of element=w389:i32)  [unwired: 1 in]
        n180 = case shown="1" w389 {
          tunnel: "预设分辨率" -> [w399 _]
          tunnel: w394 -> [w398 w460]
          frame 0, Default {
            n181 = case shown="\"分辨率2\"" w399 {
              tunnel: w398 -> [w400 w419 w420 w430 w440 w450]
              frame "分辨率1", Default {
                n182 = dll-call lib="MVCAMSDK.dll" fn="CameraSetImageResolutionEx"("相机句柄"=w400, "预设分辨率索引"=0, "Mode"=0, "ModeSize"=u32 0, "x"=0, "y"=u32 0 ("ModeSize"), "width"=0, "height"=0, "ZoomWidth"=0, "ZoomHeight"=0) -> ()  [unwired: 14 in, 2 out]
              }
              frame "分辨率2" {
                n183 = dll-call lib="MVCAMSDK.dll" fn="CameraSetImageResolutionEx"("相机句柄"=w419, "预设分辨率索引"=1, "Mode"=0, "ModeSize"=u32 0, "x"=0, "y"=u32 0 ("ModeSize"), "width"=0, "height"=0, "ZoomWidth"=0, "ZoomHeight"=0) -> ()  [unwired: 14 in, 2 out]
              }
              frame "分辨率3" {
                n184 = dll-call lib="MVCAMSDK.dll" fn="CameraSetImageResolutionEx"("相机句柄"=w420, "预设分辨率索引"=2, "Mode"=0, "ModeSize"=u32 0, "x"=0, "y"=u32 0 ("ModeSize"), "width"=0, "height"=0, "ZoomWidth"=0, "ZoomHeight"=0) -> ()  [unwired: 14 in, 2 out]
              }
              frame "分辨率4" {
                n185 = dll-call lib="MVCAMSDK.dll" fn="CameraSetImageResolutionEx"("相机句柄"=w430, "预设分辨率索引"=3, "Mode"=0, "ModeSize"=u32 0, "x"=0, "y"=u32 0 ("ModeSize"), "width"=0, "height"=0, "ZoomWidth"=0, "ZoomHeight"=0) -> ()  [unwired: 14 in, 2 out]
              }
              frame "分辨率5" {
                n186 = dll-call lib="MVCAMSDK.dll" fn="CameraSetImageResolutionEx"("相机句柄"=w440, "预设分辨率索引"=4, "Mode"=0, "ModeSize"=u32 0, "x"=0, "y"=u32 0 ("ModeSize"), "width"=0, "height"=0, "ZoomWidth"=0, "ZoomHeight"=0) -> ()  [unwired: 14 in, 2 out]
              }
              frame "分辨率6" {
                n187 = dll-call lib="MVCAMSDK.dll" fn="CameraSetImageResolutionEx"("相机句柄"=w450, "预设分辨率索引"=5, "Mode"=0, "ModeSize"=u32 0, "x"=0, "y"=u32 0 ("ModeSize"), "width"=0, "height"=0, "ZoomWidth"=0, "ZoomHeight"=0) -> ()  [unwired: 14 in, 2 out]
              }
            }
          }
          frame 1 {
            n188 = Unbundle("ROI分辨率") -> ("水平偏移"=w462:dbl, "垂直偏移"=w463:dbl, "宽度"=w464:dbl, "高度"=w465:dbl)
            n189 = dll-call lib="MVCAMSDK.dll" fn="CameraSetImageResolutionEx"("相机句柄"=w460, "预设分辨率索引"=255, "Mode"=0, "ModeSize"=u32 0, "x"=w462, "y"=w463, "width"=w464, "height"=w465, "ZoomWidth"=0, "ZoomHeight"=u32 0 ("ModeSize")) -> ()  [unwired: 14 in, 2 out]
          }
        }
      }
      event "Stop": Value Change {
        # "反初始化相机"
        n190 = event-data() -> ()  [unwired: 1 in, 6 out]
        n191 = dll-call lib="MVCAMSDK.dll" fn="CameraUnInit"("相机句柄"=w474) -> ()  [unwired: 5 in, 2 out]
      }
    }
    n192 = local write "软触发一帧"(w52) -> ()
    n193 = local write "连续模式"(w52) -> ()
    n194 = local write "自动曝光模式"(w52) -> ()
    n195 = local write "硬触发模式"(w52) -> ()
    n196 = local write "手动曝光模式"(w52) -> ()
    n197 = local write "软触发模式"(w52) -> ()
    n198 = local write "相机参数"(w52) -> ()
    n199 = Stop(stop? (T)=w48) -> ()
  }
  n200 = VISA Close(VISA resource name=w3) -> ()  [unwired: 1 in, 1 out]
